vi "move.vi"(8 "error in (no error)":errorcluster, 11 "DL090409StageScaffold in":refnum<class "StageDL090409Scaffold.lvclass">) -> (0 "error out":errorcluster, 3 "DL090409StageScaffold out":refnum<class "StageDL090409Scaffold.lvclass">)   [LabVIEW 2010, in "StageDL090409Scaffold.lvclass"]
uses:
  StageDL090409Scaffold.lvclass
  GenericStage/GenericStage/translation_mode_enum.ctl
  GenericStage/GenericStage/GenericStage.lvclass
  common/classes/SpaceVector/SpaceVector/SpaceVector.lvclass
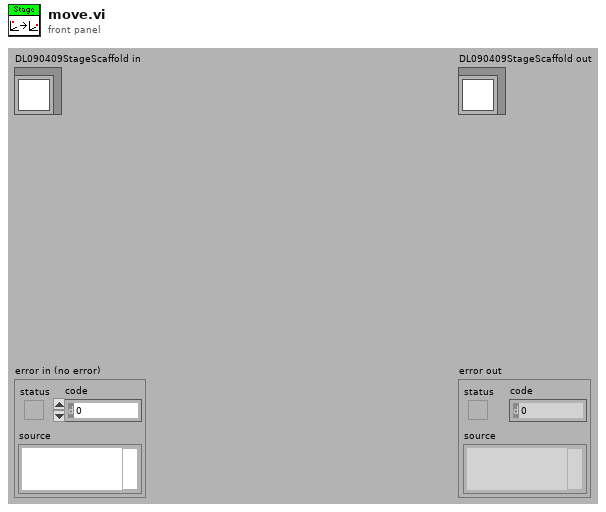
[diagram p1: front panel]
types:
  T1 = typedef "GenericStage.lvclass/translation_mode_enum.ctl" = enum16{"DON'T MOVE", "relative", "absolute"}
  T2 = typedef "GenericStage.lvclass/translation_request.ctl" = cluster{"translation mode":T1, "translation vector":refnum<class "SpaceVector.lvclass">}
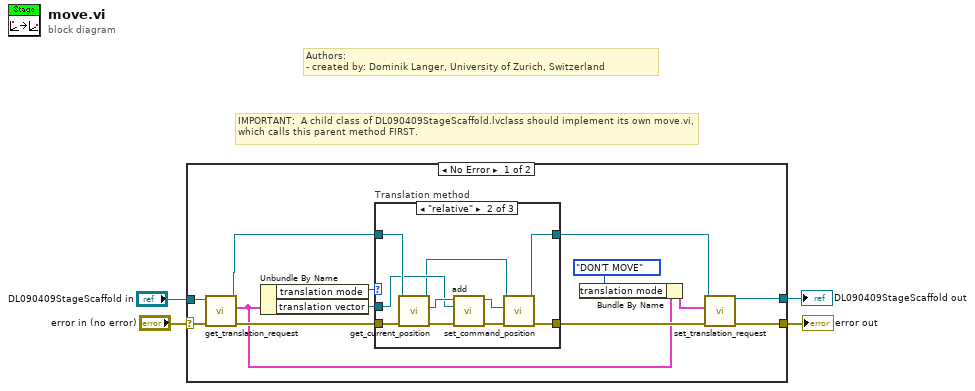
[diagram p0: block diagram]
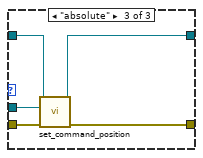
[diagram p3: hidden frame]
diagram:
  # "IMPORTANT:  A child class of DL090409StageScaffold.lvclass should implement its own move.vi, which calls this parent method FIRST."
  # "Authors: \n- created by: Dominik Langer, University of Zurich, Switzerland"
  n1 = case shown="No Error" "error in (no error)" {
    selector: "error in (no error)" -> [w17 w36]
    tunnel: [w16 w36] -> w3
    tunnel: [w15 w35] -> w1
    tunnel: "DL090409StageScaffold in" -> [w12 w35]
    frame No Error {
      n2 = call-dynamic "get_translation_request.vi"("error in (no error)"=w17, "GenericStage.lvclass in"=w12) -> ("error out"=w9:errorcluster, "translation request"=w5:T2, "GenericStage.lvclass out"=w10:refnum<class "StageDL090409Scaffold.lvclass">)  [unwired: 7 out]
      n3 = Unbundle By Name(w5) -> ("translation mode"=w11:T1, "translation vector"=w8:refnum<class "SpaceVector.lvclass">)
      n4 = case "Translation method" shown="\"relative\"" w11 {
        tunnel: w10 -> [w18 w28 w31]
        tunnel: w9 -> [w19 w29 w34]
        tunnel: w8 -> [_ w25 w32]
        tunnel: [w19 w23 w33] -> w7
        tunnel: [w18 w20 w30] -> w6
        frame "DON'T MOVE", Default {
        }
        frame "relative" {
          n5 = call-dynamic "get_current_position.vi"("error in (no error)"=w29, "DL090409StageScaffold.lvclass in"=w28) -> ("error out"=w27:errorcluster, "current position"=w26:refnum<class "SpaceVector.lvclass">, "DL090409StageScaffold.lvclass out"=w21:refnum<class "StageDL090409Scaffold.lvclass">)  [unwired: 7 out]
          n6 = call "add.vi"("error in (no error)"=w27, "vector to be added"=w25, "SpaceVector in"=w26) -> ("error out"=w24:errorcluster, "SpaceVector out"=w22:refnum<class "SpaceVector.lvclass">)  [unwired: 7 out]
          n7 = call-dynamic "set_command_position.vi"("error in (no error)"=w24, "command position"=w22, "DL090409StageScaffold.lvclass in"=w21) -> ("error out"=w23:errorcluster, "DL090409StageScaffold.lvclass out"=w20:refnum<class "StageDL090409Scaffold.lvclass">)  [unwired: 7 out]
        }
        frame "absolute" {
          n8 = call-dynamic "set_command_position.vi"("error in (no error)"=w34, "command position"=w32, "DL090409StageScaffold.lvclass in"=w31) -> ("error out"=w33:errorcluster, "DL090409StageScaffold.lvclass out"=w30:refnum<class "StageDL090409Scaffold.lvclass">)  [unwired: 7 out]
        }
      }
      n9 = Bundle By Name(cluster=w5, "translation mode"=translation_mode_enum."DON'T MOVE") -> (w14:T2)
      n10 = call-dynamic "set_translation_request.vi"("error in (no error)"=w7, "translation request"=w14, "GenericStage.lvclass in"=w6) -> ("error out"=w16:errorcluster, "GenericStage.lvclass out"=w15:refnum<class "StageDL090409Scaffold.lvclass">)  [unwired: 7 out]
    }
    frame Error {
    }
  }
  "error out" <- w3
  "DL090409StageScaffold out" <- w1
